vi "Actualiza Tabla.vi"(8 "error in (no error)":errorcluster, 10 "ACTUALIZA TABLA":bool, 11 "REFRESCOS Y PAPAS ACTOR in":refnum<class "REFRESCOS Y PAPAS ACTOR.lvclass">) -> (0 "error out":errorcluster, 3 "REFRESCOS Y PAPAS ACTOR out":refnum<class "REFRESCOS Y PAPAS ACTOR.lvclass">)   [LabVIEW 2019, in "REFRESCOS Y PAPAS ACTOR.lvlib" / "REFRESCOS Y PAPAS ACTOR.lvclass"]
uses:
  REFRESCOS Y PAPAS ACTOR.lvclass
  REFRESCOS Y PAPAS ACTOR.lvclass/REFRESCOS Y PAPAS ACTOR.ctl
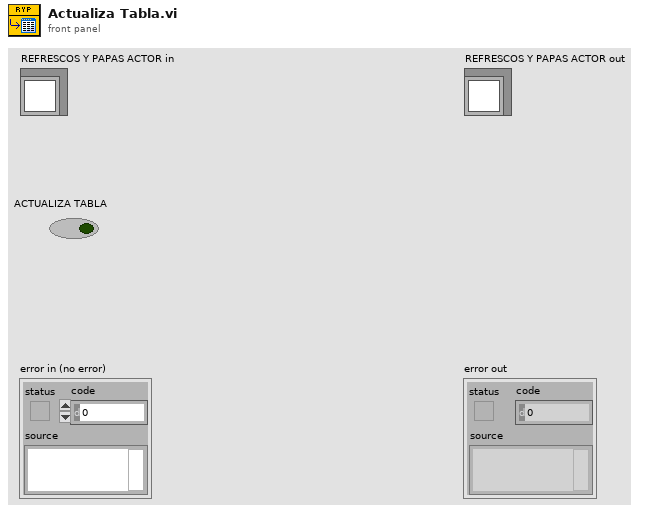
[diagram p1: front panel]
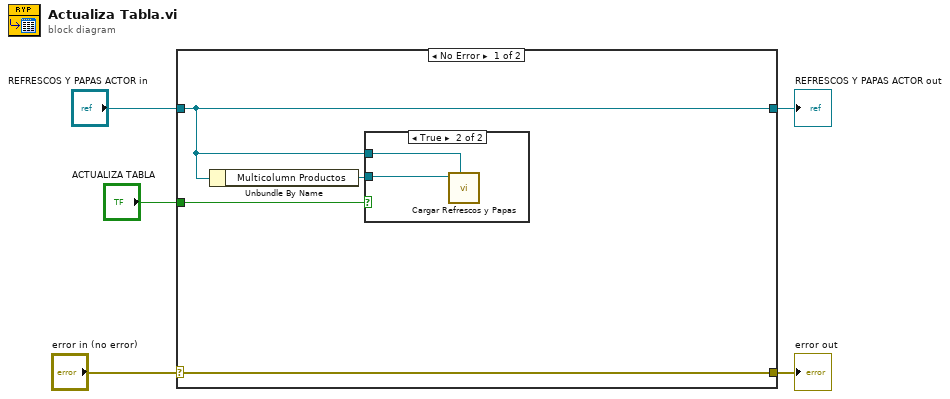
[diagram p0: block diagram]
diagram:
  n1 = case shown="No Error" "error in (no error)" {
    selector: "error in (no error)" -> [w9 w13]
    tunnel: [w9 w13] -> w4
    tunnel: [w6 w12] -> w2
    tunnel: "REFRESCOS Y PAPAS ACTOR in" -> [w6 w12]
    tunnel: "ACTUALIZA TABLA" -> [w8 _]
    frame No Error {
      n2 = Unbundle By Name(w6) -> ("Multicolumn Productos"=w7:refnum<vi>)
      n3 = case shown="True" w8 {
        tunnel: w7 -> [_ w11]
        tunnel: w6 -> [_ w10]
        frame False {
        }
        frame True {
          n4 = call "Cargar Refrescos y Papas.vi"("REFRESCOS Y PAPAS ACTOR in"=w10, "MulticolumnListbox in"=w11) -> ()  [unwired: 10 in]
        }
      }
    }
    frame Error {
    }
  }
  "error out" <- w4
  "REFRESCOS Y PAPAS ACTOR out" <- w2
